vi "effective_angle_correction.vi"(8 "orig vel calib values":dbl[][](array[numeric])=[[0.0, 0.2, 0.0, 0.0, 0.0], [1.0, 1.22, 1.0, 4.0, 5.0], [1.2, 2.24, 2.0, 4.2, 5.2], [0.0, 3.26, 3.0, 0.0, 0.0], [0.0, 4.28, 4.0, 0.0, 0.0], [0.0, 5.3, 5.0, 0.0, 0.0]] format="%.2f", 9 "angle calib values":dbl[][](array[numeric])=[[-10.0, 3.8, 4.1, 0.0, 0.0], [-5.0, 3.9, 4.05, -1.0, -2.0], [0.0, 4.0, 4.0, 2.0, 3.0], [5.0, 4.05, 3.9, 0.0, 0.0], [10.0, 4.1, 3.8, 0.0, 0.0]] format="%.2f", 11 "vel calib values":dbl[][](array[numeric])=[[0.0, 0.1, 0.0, 0.0, 0.0], [1.0, 1.11, 1.0, 4.0, 5.0], [2.0, 2.12, 2.0, 4.1, 5.1], [0.0, 3.13, 3.0, 0.0, 0.0], [0.0, 4.14, 4.0, 0.0, 0.0], [0.0, 5.15, 5.0, 0.0, 0.0]] format="%.3f") -> (3 "delta psi":dbl format="%.2f")   [LabVIEW 2010]
uses:
  <vilib>/Analysis/NI_AALPro.lvlib
panel:
  out "psi v0":dbl=9.21126429329161 format="%.2f"
  out "psi v":dbl=4.637549367807797 format="%.2f"
  out "Bv0":dbl=-19.999999999999773 format="%.2f"
  out "Av0":dbl=100.99999999999909 format="%.2f"
  out "Bv":dbl=-20.000000000000004 format="%.2e"
  out "Av":dbl=201.0 format="%.2f"
  out "Ba":dbl=7.982857142857143 format="%.2f"
  out "Aa":dbl=-0.9523809523809749 format="%.2f"
  out "?":cluster{"Best Fit":dbl[], dbl[]}[](graph)=[{"Best Fit"=[-0.2999999999999998, -0.1499999999999999, 0.0, 0.1499999999999999, 0.2999999999999998], [7.8999999999999995, 7.949999999999999, 8.0, 7.949999999999999, 7.8999999999999995]}, {"Best Fit"=[0.1, 0.1100000000000001, 0.1200000000000001, 0.1299999999999999, 0.13999999999999968, 0.15000000000000036], [0.1, 2.1100000000000003, 4.12, 6.13, 8.14, 10.15]}, {"Best Fit"=[0.2, 0.21999999999999997, 0.2400000000000002, 0.2599999999999998, 0.28000000000000025, 0.2999999999999998], [0.2, 2.2199999999999998, 4.24, 6.26, 8.280000000000001, 10.3]}, {"Best Fit"=[-0.2999999999999998, -0.1499999999999999, 0.0, 0.1499999999999999, 0.2999999999999998], [7.897142857142855, 7.961428571428571, 7.982857142857143, 7.961428571428571, 7.897142857142855]}, {"Best Fit"=[0.1, 0.1100000000000001, 0.1200000000000001, 0.1299999999999999, 0.13999999999999968, 0.15000000000000036], [0.09999999999999787, 2.110000000000017, 4.120000000000019, 6.129999999999974, 8.139999999999933, 10.150000000000066]}, {"Best Fit"=[0.2, 0.21999999999999997, 0.2400000000000002, 0.2599999999999998, 0.28000000000000025, 0.2999999999999998], [0.20000000000004547, 2.2200000000000237, 4.24000000000003, 6.25999999999997, 8.279999999999998, 10.299999999999937]}]
  out "Xv0":dbl=0.27633792879874813 format="%.2f"
  out "Xv":dbl=0.13912648103423378 format="%.3f"
  # "Yv"
  # "Yv0"
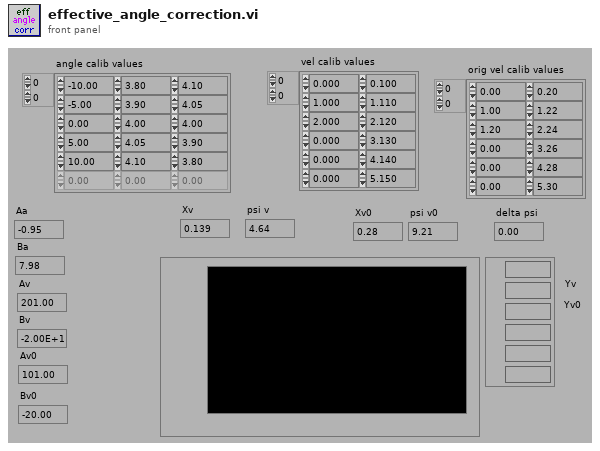
[diagram p1: front panel]
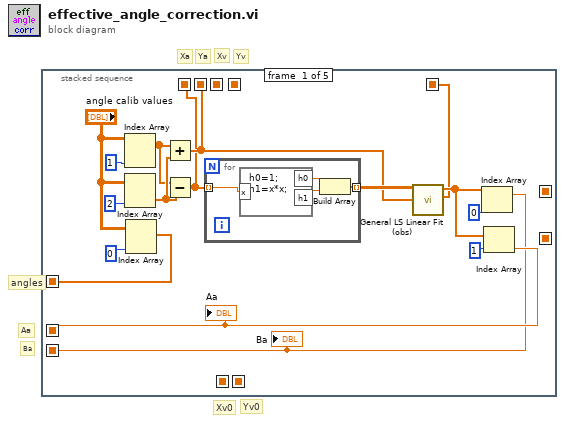
[diagram p0: block diagram]
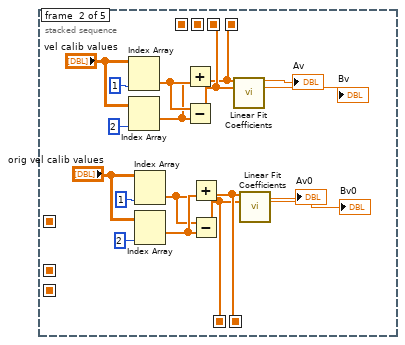
[diagram p2: hidden frame]
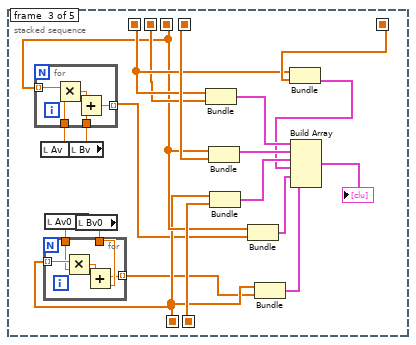
[diagram p3: hidden frame]
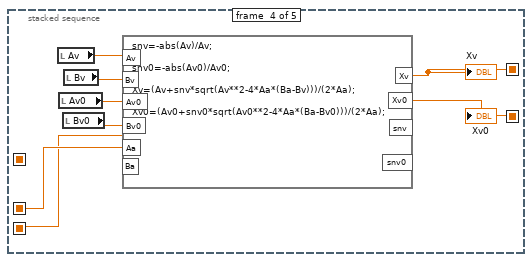
[diagram p4: hidden frame]
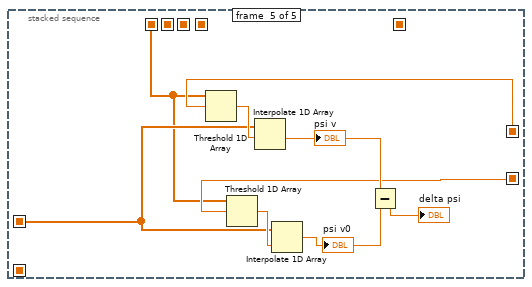
[diagram p5: hidden frame]
diagram:
  # "angles"
  # "Yv0"
  # "Xv0"
  # "Yv"
  # "Xv"
  # "Ya"
  # "Xa"
  # "Ba"
  # "Aa"
  n1 = stacked-sequence {
    seq-local: [w3 _ _ _ _] -> [_ _ _ w72 _]
    seq-local: [w2 _ _ _ _] -> [_ _ _ w71 _]
    seq-local: [w1 _ _ _ _] -> [_ _ w47 _ w79]
    seq-local: [w8 _ _ _ _] -> [_ _ w46 _ _]
    seq-local: [_ w28 _ _ _] -> [_ _ w44 _ _]
    seq-local: [_ w22 _ _ _] -> [_ _ w58 _ _]
    seq-local: [_ w21 _ _ _] -> [_ _ w43 _ _]
    seq-local: [_ w27 _ _ _] -> [_ _ w57 _ _]
    seq-local: [w5 _ _ _ _] -> [_ _ _ _ w81]
    seq-local: [w4 _ _ _ _] -> [_ _ w48 _ _]
    seq-local: [_ _ _ w70 _] -> [_ _ _ _ w84]
    seq-local: [_ _ _ w69 _] -> [_ _ _ _ w80]
    frame #0 {
      n2 = Index Array(array="angle calib values", index (col)=1) -> (element=w12:dbl[])  [unwired: 1 in]
      n3 = Index Array(array="angle calib values", index (col)=2) -> (element=w13:dbl[])  [unwired: 1 in]
      n4 = Index Array(array="angle calib values", index (col)=0) -> (element=w5:dbl[])  [unwired: 1 in]
      n5 = Add(x=w12, y=w13) -> (x+y=w8:dbl[])
      n6 = Subtract(x=w12, y=w13) -> (x-y=w1:dbl[])
      n7 = for {
        tunnel: [w18] -> w16 mode=indexing
        tunnel: w1 -> [w17] mode=indexing
        n8 = formula code="h0=1;\nh1=x*x;"("x"=w17) -> ("h0"=w20:dbl, "h1"=w19:dbl)
        n9 = Build Array(w20, w19) -> (w18:dbl[])
      }
      n10 = call <vilib>:"General LS Linear Fit (obs).vi"("H"=w16, "Y"=w8) -> ("Coefficients"=w11:dbl[], "Best Fit"=w4:dbl[])  [unwired: 3 in, 3 out]
      n11 = Index Array(array=w11, index=0) -> (element=w2:dbl)
      "Ba" <- w2
      n12 = Index Array(array=w11, index=1) -> (element=w3:dbl)
      "Aa" <- w3
    }
    frame #1 {
      n13 = Index Array(array="vel calib values", index (col)=1) -> (element=w35:dbl[])  [unwired: 1 in]
      n14 = Index Array(array="vel calib values", index (col)=2) -> (element=w34:dbl[])  [unwired: 1 in]
      n15 = Index Array(array="orig vel calib values", index (col)=1) -> (element=w32:dbl[])  [unwired: 1 in]
      n16 = Index Array(array="orig vel calib values", index (col)=2) -> (element=w33:dbl[])  [unwired: 1 in]
      n17 = Add(x=w35, y=w34) -> (x+y=w22:dbl[])
      n18 = Subtract(x=w35, y=w34) -> (x-y=w28:dbl[])
      n19 = Add(x=w32, y=w33) -> (x+y=w27:dbl[])
      n20 = Subtract(x=w32, y=w33) -> (x-y=w21:dbl[])
      n21 = call <vilib>:"Linear Fit Coefficients.vi"("Y"=w22, "X"=w28) -> ("slope"=→"Av":dbl, "intercept"=→"Bv":dbl)  [unwired: 11 in, 1 out]
      n22 = call <vilib>:"Linear Fit Coefficients.vi"("Y"=w27, "X"=w21) -> ("slope"=→"Av0":dbl, "intercept"=→"Bv0":dbl)  [unwired: 11 in, 1 out]
    }
    frame #2 {
      n23 = local read "Av"() -> (w51:dbl)
      n24 = local read "Av0"() -> (w41:dbl)
      n25 = local read "Bv"() -> (w45:dbl)
      n26 = for {
        tunnel: w44 -> [w68] mode=indexing
        tunnel: w51 -> [w67]
        tunnel: w45 -> [w65]
        tunnel: [w64] -> w40 mode=indexing
        n27 = Multiply(x=w68, y=w67) -> (x*y=w66:dbl)
        n28 = Add(x=w66, y=w65) -> (x+y=w64:dbl)
      }
      n29 = local read "Bv0"() -> (w42:dbl)
      n30 = for {
        tunnel: w43 -> [w63] mode=indexing
        tunnel: [w59] -> w39 mode=indexing
        tunnel: w42 -> [w62]
        tunnel: w41 -> [w61]
        n31 = Multiply(x=w63, y=w61) -> (x*y=w60:dbl)
        n32 = Add(x=w60, y=w62) -> (x+y=w59:dbl)
      }
      n33 = Bundle(w47, w46) -> (w56:cluster{dbl[], dbl[]})  [unwired: 1 in]
      n34 = Bundle(w44, w58) -> (w55:cluster{dbl[], dbl[]})  [unwired: 1 in]
      n35 = Bundle(w43, w57) -> (w54:cluster{dbl[], dbl[]})  [unwired: 1 in]
      n36 = Bundle(w44, w40) -> (w50:cluster{dbl[], dbl[]})  [unwired: 1 in]
      n37 = Bundle(w43, w39) -> (w49:cluster{dbl[], dbl[]})  [unwired: 1 in]
      n38 = Bundle(w47, "Best Fit"=w48) -> (w52:cluster{dbl[], "Best Fit":dbl[]})  [unwired: 1 in]
      n39 = Build Array(w56, w55, w54, w52, w50, w49) -> (→"?":cluster{dbl[], "Best Fit":dbl[]}[])
    }
    frame #3 {
      n40 = local read "Av"() -> (w76:dbl)
      n41 = local read "Av0"() -> (w74:dbl)
      n42 = local read "Bv0"() -> (w73:dbl)
      n43 = local read "Bv"() -> (w75:dbl)
      n44 = formula code="snv=-abs(Av)/Av;\n\nsnv0=-abs(Av0)/Av0;\n\nXv=(Av+snv*sqrt(Av**2-4*Aa*(Ba-Bv)))/(2*Aa);\n\nXv0=(Av0+snv0*sqrt(Av0**2-4*Aa*(Ba-Bv0)))/(2*Aa);"("Av"=w76, "Bv"=w75, "Av0"=w74, "Bv0"=w73, "Aa"=w72, "Ba"=w71) -> ("Xv"=w70:dbl, "Xv0"=w69:dbl)  [unwired: 2 out]
      "Xv" <- w70
      "Xv0" <- w69
    }
    frame #4 {
      n45 = Threshold 1D Array(2:w84, 3:w79) -> (0:w85:dbl)  [unwired: 1 in]
      n46 = Threshold 1D Array(2:w80, 3:w79) -> (0:w82:dbl)  [unwired: 1 in]
      n47 = Interpolate 1D Array(1:w85, 2:w81) -> (0:w83:dbl)
      "psi v" <- w83
      n48 = Interpolate 1D Array(1:w82, 2:w81) -> (0:w78:dbl)
      "psi v0" <- w78
      n49 = Subtract(x=w83, y=w78) -> (x-y=→"delta psi":dbl)
    }
  }
